vi "Test Copy Image No Mask Greyscale.vi"(8 "error in (no error)":errorcluster, 11 "Test Case In":refnum<class "01_Image.lvclass">) -> (0 "error out":errorcluster, 3 "Test Case Out":refnum<class "01_Image.lvclass">)   [LabVIEW 2020, in "test.lvlib" / "01_Image.lvclass"]
uses:
  01_Image.lvclass
  C:/Program Files (x86)/National Instruments/LabVIEW 2026/vi.lib/Astemes/LUnit/Test Case.lvclass
  common/Image Size (Integer).ctl
  <vilib>/Astemes/LUnit/Test Case.lvclass/Test Case.ctl
  image/New Image (Greyscale Preallocated).vi
  image/Copy Image (Greyscale).vi
  4993e8ee-a06a-463a-9684-69129f64d5ce.vi
  image/Copy Array to Image.vi
  image/Copy Array to Image (Greyscale).vi
  image/New Image (Greyscale Preallocated).vi/6598b9e0-8a08-46f5-91fd-ca1b87217137.vi
  image/Copy Image (Greyscale).vi/c92252ab-1097-45af-a449-7a3c8cf05290.vi
  <vilib>/Astemes/LUnit/Core/LUnit Test Case/Private/Append Pass Result.vi
  <vilib>/Astemes/LUnit/Core/LUnit Test Case/Private/Append Fail Result.vi
  4993e8ee-a06a-463a-9684-69129f64d5ce.vi/9c5d11cd-9439-4240-a1ee-d9baace9c924.vi
  <vilib>/Astemes/LUnit/Core/LUnit Test Case/Private/Run In UI.vi
  <vilib>/Utility/error.llb/Clear Errors.vi
  <vilib>/Utility/error.llb/Error Cluster From Error Code.vi
  <vilib>/picture/pixmap.llb/Flatten Pixmap.vi
  image/image.lvlib
  common/common.lvlib
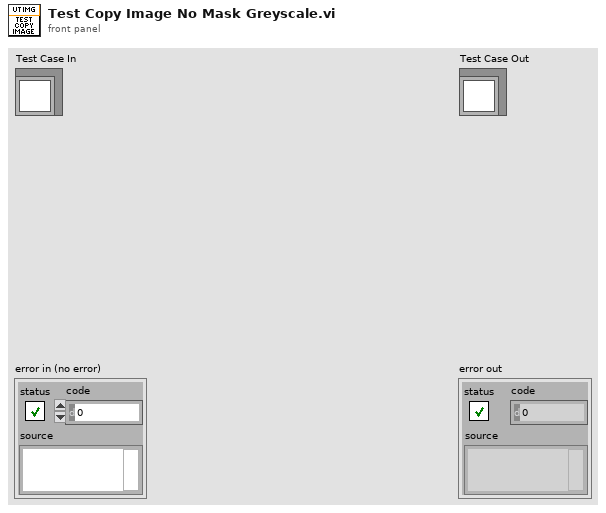
[diagram p1: front panel]
types:
  T1 = typedef "common.lvlib/Image Size (Integer).ctl" = cluster{"Width":u16, "Height":u16}
  T2 = typedef "image.lvlib/Greyscale Image.ctl" = refnum<data-value>
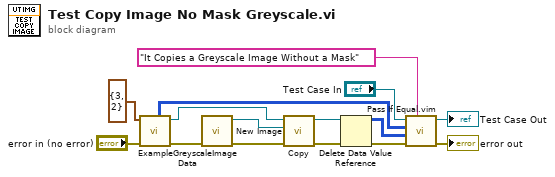
[diagram p0: block diagram]
diagram:
  n1 = call "ExampleGreyscaleImageData.vi"("error in (no error)"="error in (no error)", "Image Size"=T1 {"Width"=3, "Height"=2}) -> ("error out"=w3:errorcluster, "Greyscale Destination Image"=w1:T2, "Greyscale Data"=w6:u8[][])  [unwired: 6 in, 1 out]
  n2 = call-poly "New Image.vi"("error in (no error)"=w3) -> ("error out"=w11:errorcluster, "Greyscale Image"=w5:T2)  [unwired: 9 in]
  n3 = call-poly "Copy.vi"("error in (no error)"=w11, "Greyscale Image Destination in"=w5, "Greyscale Image Source in"=w1) -> ("error out"=w9:errorcluster, "Greyscale Image Destination"=w8:T2)  [unwired: 7 in]
  n4 = Delete Data Value Reference(data value reference=w8, error in=w9) -> (data value=w7:u8[][], error out=w10:errorcluster)
  n5 = call "Pass If Equal.vim"("Description"="It Copies a Greyscale Image Without a Mask", "error in (no error)"=w10, "Actual"=w7, "Expected"=w6, "LUnit Test Case In"="Test Case In") -> ("error out"=→"error out":errorcluster, "LUnit Test Case Out"=→"Test Case Out":refnum<class "01_Image.lvclass">)  [unwired: 5 in]
